vi "TCP Listener.vi"() -> ()   [LabVIEW 2019]
panel:
  out "No of messages":i32
  out "Recieved Messages":string[](array[string])
  out "Current Message":string
  in  "error in (no error)":errorcluster
  out "error out":errorcluster
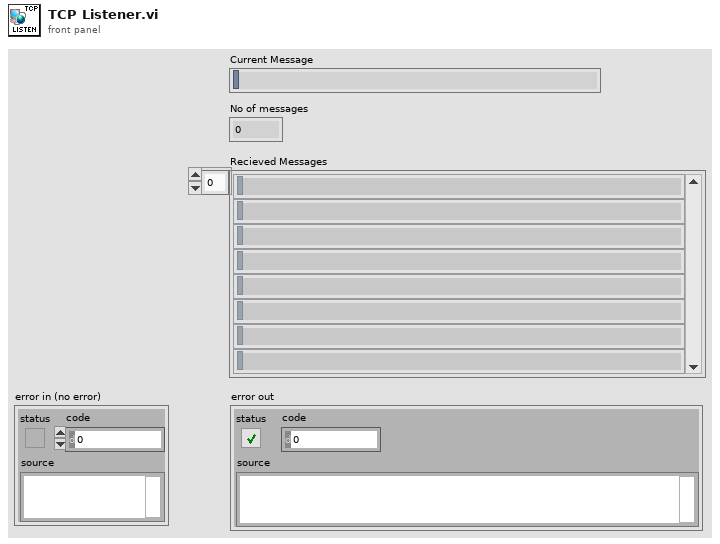
[diagram p1: front panel]
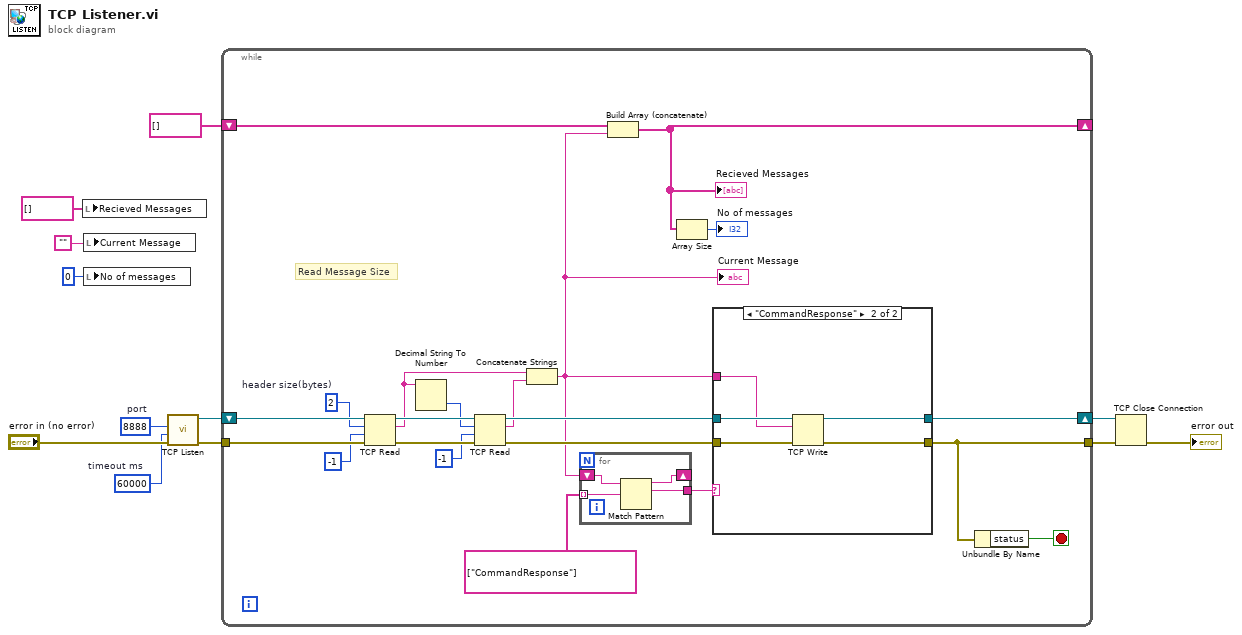
[diagram p0: block diagram]
diagram:
  w4 = 60000  # timeout ms
  w9 = u16 8888  # port
  n1 = local write "Recieved Messages"(string[] [] ("Recieved Messages")) -> ()
  n2 = local write "Current Message"("") -> ()
  n3 = local write "No of messages"(0 ("No of messages")) -> ()
  n4 = call <vilib>:"TCP Listen.vi"("error in (no error)"="error in (no error)", "timeout ms (wait forever: -1)"=w4, "port"=w9) -> ("error out"=w7:errorcluster, "connection ID"=w8:refnum<k5>)  [unwired: 4 in, 3 out]
  n5 = while {
    shift-right: [w18] -> _
    shift-left: string[] [] -> [w31]
    shift-right: [w20] -> w12
    shift-left: w8 -> [w33]
    tunnel: w7 -> [w32]
    tunnel: [w22] -> w11
    stop <- w23 stop-if-true
    w30 = 2  # header size(bytes)
    # "Read Message Size"
    n6 = TCP Read(connection ID=w33, bytes to read=w30, error in (no error)=w32, 9:-1 ("timeout ms (25000)")) -> (connection ID out=w27:refnum<k5>, data out=w13:string, error out=w28:errorcluster)  [unwired: 1 in]
    n7 = Decimal String To Number(string=w13) -> (number=w26:i32)  [unwired: 2 in, 1 out]
    n8 = TCP Read(connection ID=w27, bytes to read=w26, error in (no error)=w28, 9:-1 ("timeout ms (25000)")) -> (connection ID out=w21:refnum<k5>, data out=w15:string, error out=w24:errorcluster)  [unwired: 1 in]
    n9 = Concatenate Strings(w13, w15) -> (w14:string)
    "Current Message" <- w14
    n10 = for {
      tunnel: string[] ["CommandResponse"] ("regular expression") -> [w36] mode=indexing
      tunnel: [w37] -> w17
      shift-right: [w34] -> _
      shift-left: w14 -> [w35]
      n11 = Match Pattern(string=w35, regular expression=w36) -> (before substring=w34:string, match substring=w37:string)  [unwired: 1 in, 2 out]
    }
    n12 = Build Array (concatenate)(w31, w14) -> (w18:string[])
    "Recieved Messages" <- w18
    n13 = Array Size(array=w18) -> (size(s)=→"No of messages":i32)
    n14 = case shown="\"CommandResponse\"" w17 {
      tunnel: w24 -> [w39 w44]
      tunnel: [w39 w43] -> w22
      tunnel: w21 -> [w38 w42]
      tunnel: [w38 w41] -> w20
      tunnel: w14 -> [_ w40]
      frame "CommandOnly", Default {
      }
      frame "CommandResponse" {
        n15 = TCP Write(connection ID=w42, data in=w40, error in (no error)=w44) -> (connection ID out=w41:refnum<k5>, error out=w43:errorcluster)  [unwired: 1 in, 1 out]
      }
    }
    n16 = Unbundle By Name(w22) -> ("status"=w23:bool)
  }
  n17 = TCP Close Connection(connection ID=w12, error in (no error)=w11) -> (error out=→"error out":errorcluster)  [unwired: 1 in, 1 out]
